vi "getCalib.vi"() -> ()   [LabVIEW 2013]
uses:
  lens_TypDEf.ctl
panel:
  out "output array 3":dbl[][](graph)
  out "time":u32
  out "cam2":path=path "cam2"
  in  "Numeric":i32=2
  out "output cluster":cluster{"dp [MeV/C]":dbl[], dbl[]}[](graph)
  in  "B [T]":dbl=1.0
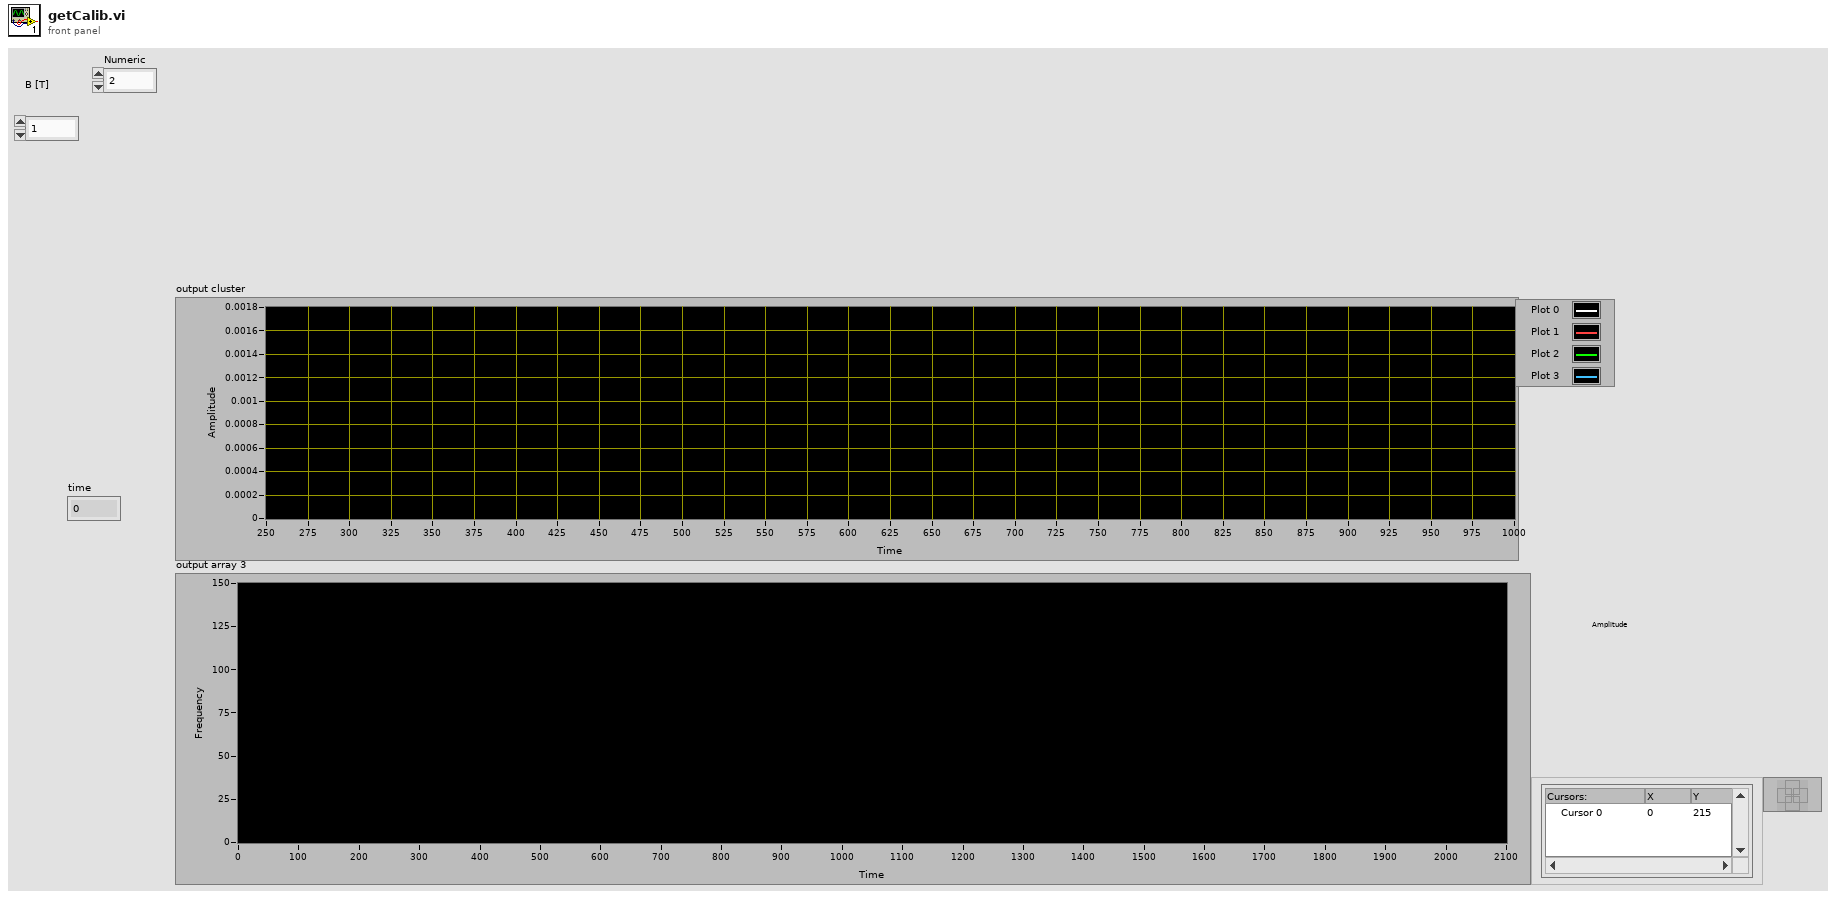
[diagram p1: front panel]
types:
  T1 = typedef "lens_TypDEf.ctl" = string
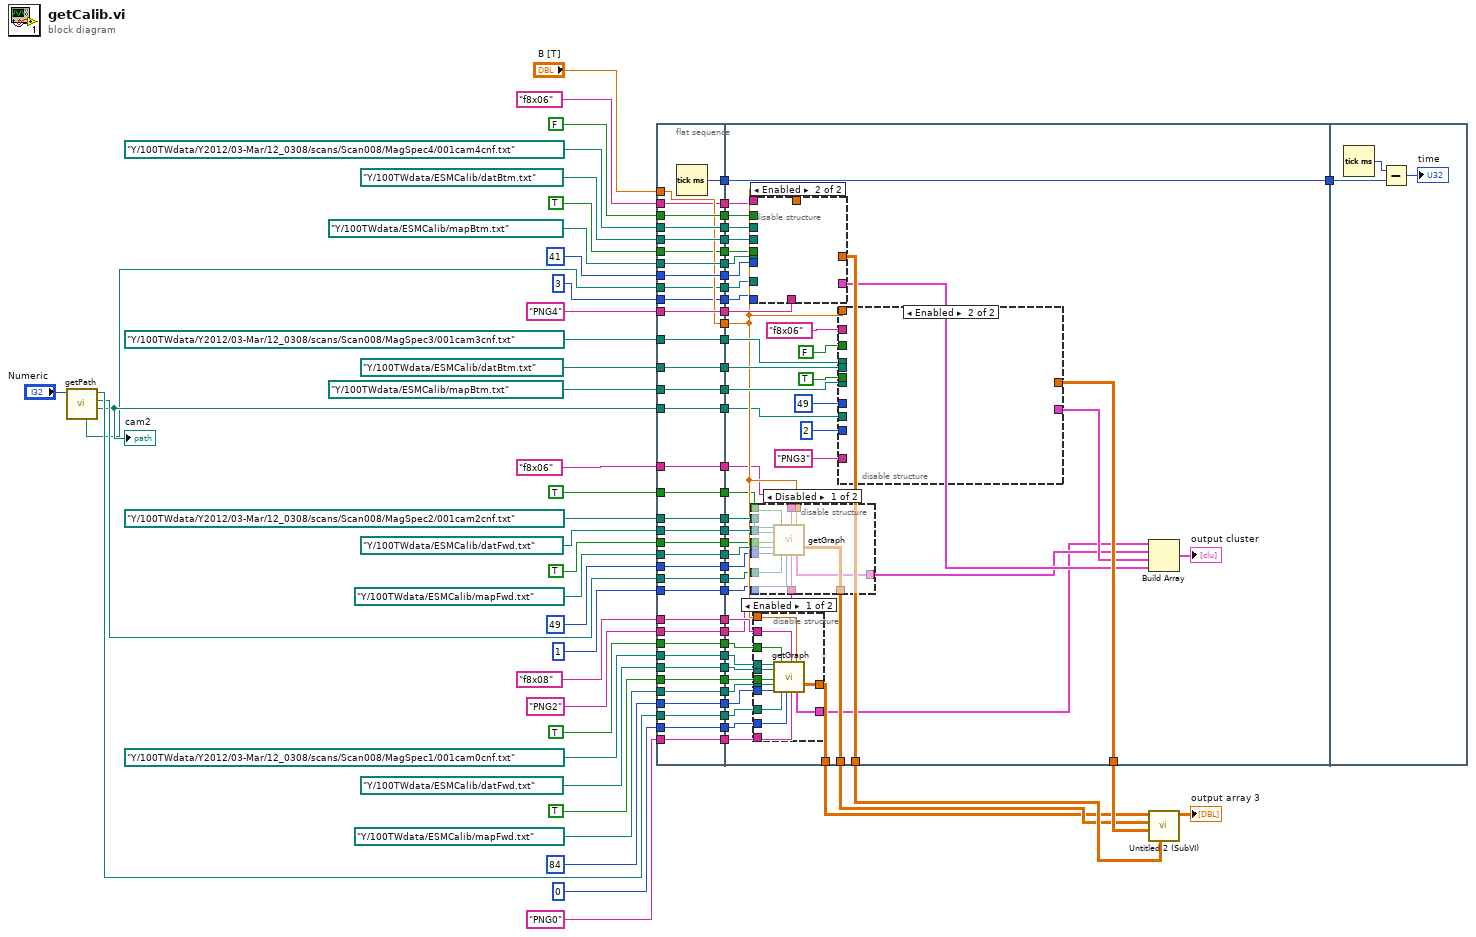
[diagram p0: block diagram]
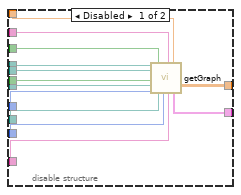
[diagram p3: hidden frame]
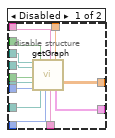
[diagram p4: hidden frame]
diagram:
  n1 = call "getPath.vi"("Numeric"="Numeric") -> ("cam2"=w44:path, "cam1"=w45:path, "cam0"=w46:path, "cam3"=w43:path)  [unwired: 7 in]
  "cam2" <- w44
  n2 = flat-sequence {
    tunnel: w43 -> [w80]
    tunnel: w44 -> [w81]
    tunnel: w45 -> [w82]
    tunnel: w46 -> [w83]
    tunnel: TRUE ("ROI") -> [w84]
    tunnel: TRUE ("ROI") -> [w85]
    tunnel: 0 ("cam (0,1,2,3)") -> [w86]
    tunnel: 1 ("cam (0,1,2,3)") -> [w87]
    tunnel: "f8x06" ("Lens") -> [w88]
    tunnel: 49 ("y0 2") -> [w89]
    tunnel: "PNG2" ("Image Name") -> [w90]
    tunnel: TRUE ("FW") -> [w91]
    tunnel: 84 ("y0") -> [w92]
    tunnel: TRUE ("FW") -> [w93]
    tunnel: "PNG0" ("Image Name") -> [w94]
    tunnel: TRUE ("ROI") -> [w95]
    tunnel: 3 ("cam (0,1,2,3)") -> [w96]
    tunnel: T1 "f8x06" ("Lens") -> [w97]
    tunnel: "f8x08" ("Lens") -> [w98]
    tunnel: "B [T]" -> [w99]
    tunnel: path "Y:/100TWdata/ESMCalib/mapFwd.txt" ("map") -> [w100]
    tunnel: path "Y:/100TWdata/ESMCalib/datFwd.txt" ("Spec_Calib_file") -> [w101]
    tunnel: path "Y:/100TWdata/Y2012/03-Mar/12_0308/scans/Scan008/MagSpec2/001cam2cnf.txt" ("Cam_Calib_file") -> [w102]
    tunnel: 41 ("y0 4") -> [w103]
    tunnel: path "Y:/100TWdata/ESMCalib/mapBtm.txt" ("map") -> [w104]
    tunnel: path "Y:/100TWdata/ESMCalib/datBtm.txt" ("Spec_Calib_file") -> [w105]
    tunnel: path "Y:/100TWdata/Y2012/03-Mar/12_0308/scans/Scan008/MagSpec4/001cam4cnf.txt" ("Cam_Calib_file") -> [w106]
    tunnel: FALSE ("FW") -> [w107]
    tunnel: "PNG4" ("Image Name") -> [w108]
    tunnel: path "Y:/100TWdata/ESMCalib/datBtm.txt" ("Spec_Calib_file") -> [w109]
    tunnel: path "Y:/100TWdata/ESMCalib/mapBtm.txt" ("map") -> [w110]
    tunnel: path "Y:/100TWdata/Y2012/03-Mar/12_0308/scans/Scan008/MagSpec3/001cam3cnf.txt" ("Cam_Calib_file") -> [w111]
    tunnel: path "Y:/100TWdata/Y2012/03-Mar/12_0308/scans/Scan008/MagSpec1/001cam0cnf.txt" ("Cam_Calib_file") -> [w112]
    tunnel: path "Y:/100TWdata/ESMCalib/datFwd.txt" ("Spec_Calib_file") -> [w113]
    tunnel: path "Y:/100TWdata/ESMCalib/mapFwd.txt" ("map") -> [w114]
    tunnel: [w114] -> w42
    tunnel: [w113] -> w41
    tunnel: [w112] -> w40
    tunnel: [w111] -> w39
    tunnel: [w110] -> w38
    tunnel: [w109] -> w37
    tunnel: [w108] -> w36
    tunnel: [w107] -> w35
    tunnel: [w106] -> w34
    tunnel: [w105] -> w33
    tunnel: [w104] -> w32
    tunnel: [w103] -> w31
    tunnel: [w102] -> w30
    tunnel: [w101] -> w29
    tunnel: [w100] -> w28
    tunnel: [w99] -> w27
    tunnel: [w98] -> w26
    tunnel: [w97] -> w25
    tunnel: [w96] -> w24
    tunnel: [w95] -> w23
    tunnel: [w94] -> w22
    tunnel: [w93] -> w21
    tunnel: [w92] -> w20
    tunnel: [w91] -> w19
    tunnel: [w90] -> w18
    tunnel: [w89] -> w17
    tunnel: [w88] -> w16
    tunnel: [w87] -> w15
    tunnel: [w86] -> w14
    tunnel: [w85] -> w13
    tunnel: [w84] -> w12
    tunnel: [w83] -> w11
    tunnel: [w82] -> w10
    tunnel: [w81] -> w9
    tunnel: [w80] -> w8
    tunnel: [w79] -> w7
    tunnel: w42 -> [w165]
    tunnel: w41 -> [w164]
    tunnel: w40 -> [w163]
    tunnel: w39 -> [w162]
    tunnel: w38 -> [w161]
    tunnel: w37 -> [w160]
    tunnel: w36 -> [w159]
    tunnel: w35 -> [w158]
    tunnel: w34 -> [w157]
    tunnel: w33 -> [w156]
    tunnel: w32 -> [w155]
    tunnel: w31 -> [w154]
    tunnel: w30 -> [w153]
    tunnel: w29 -> [w152]
    tunnel: w28 -> [w151]
    tunnel: w27 -> [w150]
    tunnel: w26 -> [w149]
    tunnel: w25 -> [w148]
    tunnel: w24 -> [w147]
    tunnel: w23 -> [w146]
    tunnel: w22 -> [w145]
    tunnel: w21 -> [w144]
    tunnel: w20 -> [w140]
    tunnel: w19 -> [w139]
    tunnel: w18 -> [w138]
    tunnel: w17 -> [w137]
    tunnel: w16 -> [w136]
    tunnel: w15 -> [w133]
    tunnel: w14 -> [w132]
    tunnel: w13 -> [w130]
    tunnel: w12 -> [w129]
    tunnel: w11 -> [w127]
    tunnel: w10 -> [w126]
    tunnel: w9 -> [w125]
    tunnel: w8 -> [w124]
    tunnel: w7 -> [w123]
    tunnel: [w123] -> w6
    tunnel: [w122] -> w5
    tunnel: [w121] -> w4
    tunnel: [w120] -> w2
    tunnel: [w119] -> w3
    tunnel: w6 -> [w219]
    frame #0 {
      n3 = Tick Count (ms)() -> (millisecond timer value=w79:u32)
    }
    frame #1 {
      n4 = disable-structure shown="Enabled" {
        disable-tunnel: w159 -> [w204 _]
        disable-tunnel: w158 -> [w203 _]
        disable-tunnel: w157 -> [w202 _]
        disable-tunnel: w156 -> [w201 _]
        disable-tunnel: w155 -> [w200 _]
        disable-tunnel: w154 -> [w199 _]
        disable-tunnel: w150 -> [w198 _]
        disable-tunnel: w148 -> [w197 _]
        disable-tunnel: w147 -> [w196 _]
        disable-tunnel: w146 -> [w195 _]
        disable-tunnel: w124 -> [w194 _]
        disable-tunnel: [w193 _] -> w122
        disable-tunnel: [w192 _] -> w118
        frame Disabled {
          n5 = call "getGraph.vi"("Cam_Calib_file"=w202, "Spec_Calib_file"=w201, "ROI"=w195, "map"=w200, "y0"=w199, "FW"=w203, "image in"=w194, "cam (0,1,2,3)"=w196, "Lens"=w197, "Image Name"=w204, "B [T]"=w198) -> ("output cluster"=w192:cluster{"dp [MeV/C]":dbl[], dbl[]}, "z"=w193:dbl[][])  [unwired: 3 in, 4 out]
        }
        frame Enabled {
        }
      }
      n6 = disable-structure shown="Disabled" {
        disable-tunnel: w153 -> [w178 _]
        disable-tunnel: w152 -> [w177 _]
        disable-tunnel: w151 -> [w176 _]
        disable-tunnel: w150 -> [w175 _]
        disable-tunnel: w139 -> [w174 _]
        disable-tunnel: w138 -> [w173 _]
        disable-tunnel: w137 -> [w172 _]
        disable-tunnel: w136 -> [w171 _]
        disable-tunnel: w133 -> [w170 _]
        disable-tunnel: w130 -> [w169 _]
        disable-tunnel: w126 -> [w168 _]
        disable-tunnel: [w167 _] -> w119
        disable-tunnel: [w166 _] -> w116
        frame Disabled {
          n7 = call "getGraph.vi"("Cam_Calib_file"=w178, "Spec_Calib_file"=w177, "ROI"=w169, "map"=w176, "y0"=w172, "FW"=w174, "image in"=w168, "cam (0,1,2,3)"=w170, "Lens"=w171, "Image Name"=w173, "B [T]"=w175) -> ("output cluster"=w166:cluster{"dp [MeV/C]":dbl[], dbl[]}, "z"=w167:dbl[][])  [unwired: 3 in, 4 out]
        }
        frame Enabled {
        }
      }
      n8 = disable-structure shown="Enabled" {
        disable-tunnel: w165 -> [w217 _]
        disable-tunnel: w164 -> [w216 _]
        disable-tunnel: w163 -> [w215 _]
        disable-tunnel: w150 -> [w214 _]
        disable-tunnel: w149 -> [w213 _]
        disable-tunnel: w145 -> [w212 _]
        disable-tunnel: w144 -> [w211 _]
        disable-tunnel: w140 -> [w210 _]
        disable-tunnel: w132 -> [w209 _]
        disable-tunnel: w129 -> [w208 _]
        disable-tunnel: w127 -> [w207 _]
        disable-tunnel: [w206 _] -> w120
        disable-tunnel: [w205 _] -> w115
        frame Enabled {
          n9 = call "getGraph.vi"("Cam_Calib_file"=w215, "Spec_Calib_file"=w216, "ROI"=w208, "map"=w217, "y0"=w210, "FW"=w211, "image in"=w207, "cam (0,1,2,3)"=w209, "Lens"=w213, "Image Name"=w212, "B [T]"=w214) -> ("output cluster"=w205:cluster{"dp [MeV/C]":dbl[], dbl[]}, "z"=w206:dbl[][])  [unwired: 3 in, 4 out]
        }
        frame Disabled {
        }
      }
      n10 = disable-structure shown="Enabled" {
        disable-tunnel: w162 -> [w191 _]
        disable-tunnel: w161 -> [w190 _]
        disable-tunnel: w160 -> [w189 _]
        disable-tunnel: w150 -> [w188 _]
        disable-tunnel: FALSE ("FW") -> [w187 _]
        disable-tunnel: "PNG3" ("Image Name") -> [w186 _]
        disable-tunnel: 49 ("y0 3") -> [w185 _]
        disable-tunnel: "f8x06" ("Lens") -> [w184 _]
        disable-tunnel: TRUE ("ROI") -> [w183 _]
        disable-tunnel: 2 ("cam (0,1,2,3)") -> [w182 _]
        disable-tunnel: w125 -> [w181 _]
        disable-tunnel: [w180 _] -> w121
        disable-tunnel: [w179 _] -> w117
        frame Disabled {
          n11 = call "getGraph.vi"("Cam_Calib_file"=w191, "Spec_Calib_file"=w189, "ROI"=w183, "map"=w190, "y0"=w185, "FW"=w187, "image in"=w181, "cam (0,1,2,3)"=w182, "Lens"=w184, "Image Name"=w186, "B [T]"=w188) -> ("output cluster"=w179:cluster{"dp [MeV/C]":dbl[], dbl[]}, "z"=w180:dbl[][])  [unwired: 3 in, 4 out]
        }
        frame Enabled {
        }
      }
      n12 = Build Array(w115, w116, w117, w118) -> (→"output cluster":cluster{"dp [MeV/C]":dbl[], dbl[]}[])
    }
    frame #2 {
      n13 = Tick Count (ms)() -> (millisecond timer value=w220:u32)
      n14 = Subtract(x=w220, y=w219) -> (x-y=→"time":u32)
    }
  }
  n15 = call "Untitled 2 (SubVI).vi"("z 4"=w5, "z 3"=w4, "z 2"=w3, "z"=w2) -> ("Array"=→"output array 3":dbl[][])  [unwired: 7 in]
